vi "Vision Example Robot Main.vi"() -> ()   [LabVIEW 2017]
doc: "This VI implements the framework and scheduler for your robotics program. It should not be necessary to modify the framework. You are expected to add your code to the VIs called from Robot Main - the ones located in the Team Code folder within the project."
uses:
  <vilib>/Rock Robotics/WPI/Camera/WPI_CameraImageSize.ctl
  Robot Global Data.vi
panel:
  in  "Image Size":T1
  in  "Enable Vision":bool=TRUE
  in  "Finish":bool
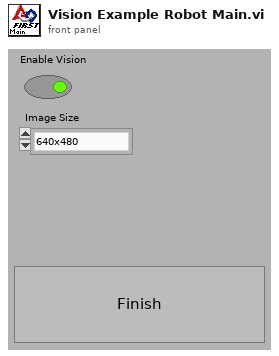
[diagram p1: front panel]
types:
  T1 = typedef "WPI_CameraImageSize.ctl" = enum16{"640x480", "320x240", "160x120", "Custom"}
  T2 = typedef "WPI_DriverStationMatch Info.ctl" = cluster{"Autonomous Elapsed Seconds":dbl, "TeleOp Elapsed Seconds":dbl, "Disabled Elapsed Seconds":dbl, "Visited Autonomous":bool, "Visited TeleOp":bool, "Visited Disabled":bool, "Autonomous Settings":cluster{"Autonomous Style":enum16{"Iterative", "Independent"}, "VI Refnum":refnum<vi>}}
  T3 = typedef "WPI_DriverStationDerivedRobotMode.ctl" = enum16{"Init", "Execute", "Stop"}
  T4 = typedef "WPI_DriverStationRobotMode2.ctl" = enum16{"Autonomous Disabled", "Autonomous Enabled", "Teleop Disabled", "Teleop Enabled", "Disconnected", "Finish", "Test Disabled", "Test Enabled", "Emergency Stopped"}
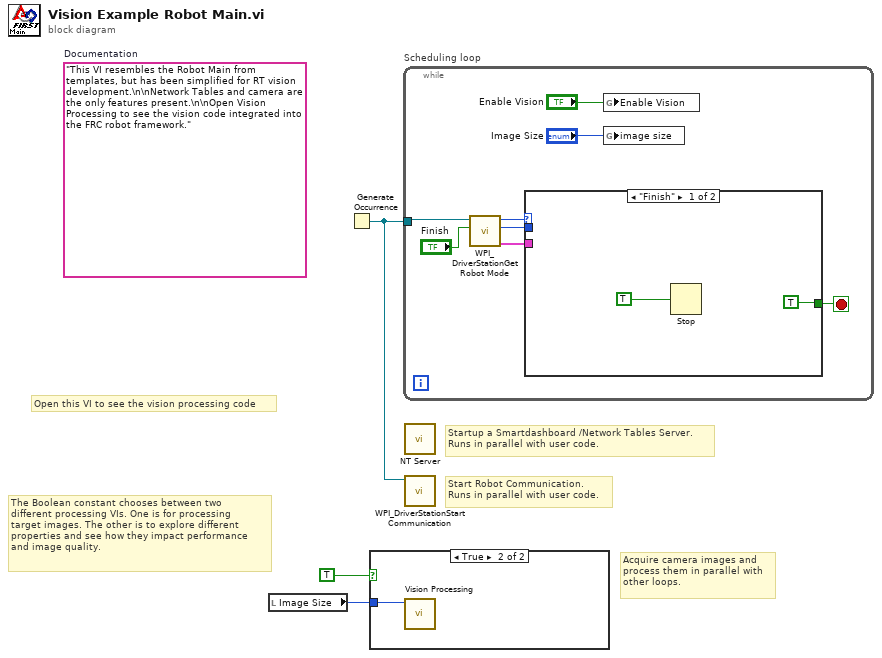
[diagram p0: block diagram]
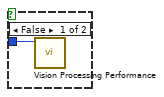
[diagram p2: hidden frame]
diagram:
  (unwired) "This VI resembles the Robot Main from templates, but has been simplified for RT vision development.\n\nNetwork Tables and camera are the only features present.\n\nOpen Vision Processing to see the vision code integrated into the FRC robot framework."  # Documentation
  # "The Boolean constant chooses between two\ndifferent processing VIs. One is for processing\ntarget images. The other is to explore different\nproperties and see how they impact performance\nand image quality."
  # "Open this VI to see the vision processing code"
  # "Startup a Smartdashboard /Network Tables Server.\nRuns in parallel with user code."
  # "Acquire camera images and\nprocess them in parallel with\nother loops."
  # "Start Robot Communication.\nRuns in parallel with user code."
  n1 = local read "Image Size"() -> (w2:T1)
  n2 = Generate Occurrence() -> (w3:refnum<k4>)
  n3 = case shown="True" TRUE {
    tunnel: w2 -> [w4 w5]
    frame False {
      n4 = call "Vision Processing Performance.vi"("Image Size"=w4) -> ()  [unwired: 7 in]
    }
    frame True {
      n5 = call "Vision Processing.vi"("Image Size"=w5) -> ()  [unwired: 11 in]
    }
  }
  n6 = while "Scheduling loop" {
    tunnel: w3 -> [w12]
    stop <- w9 stop-if-true
    n7 = call <vilib>:"WPI_DriverStationGet Robot Mode.vi"("Finish"="Finish", "DS Occurrence"=w12) -> ("Match Info out"=w10:T2, "Call Context"=w13:T3, "Robot Mode"=w6:T4)  [unwired: 7 out]
    n8 = case shown="\"Finish\"" w6 {
      tunnel: w13 -> [_ _]
      tunnel: w10 -> [_ _]
      tunnel: [TRUE _] -> w9
      frame "Finish" {
        n9 = Stop(stop? (T)=TRUE ("Quit")) -> ()
      }
      frame Default {
      }
    }
    n10 = global write "Robot Global Data.vi" "Enable Vision"("Enable Vision") -> ()
    n11 = global write "Robot Global Data.vi" "image size"("Image Size") -> ()
  }
  n12 = call <vilib>:"NT Server.vi"() -> ()  [unwired: 12 in]
  n13 = call <vilib>:"WPI_DriverStationStart Communication.vi"("occurrence"=w3) -> ()  [unwired: 1 in, 10 out]
